vi "Sample Pad Example (LINX).vi"() -> ()   [LabVIEW 2020]
doc: "A simple sample pad, which can trigger up to 16 simultaneous sound effects. Demonstrates the Mixer component, including file loading, playback, and mixer audio monitoring via a music visualizer."
uses:
  Mixer/Channel/Controls/Channel State.ctl
  Mixer/Mixer/Mixer.lvclass/Mixer.ctl
  <vilib>/MakerHub/LINX/Public/Peripherals/Digital/Digital Read N Chans.vi
  e8fa8eb6-c38c-4b8a-b362-922d187964a0.vi
  <vilib>/MakerHub/LINX/Private/Local IO/LinxDigitalRead.vi
  <vilib>/MakerHub/LINX/Public/Utilities/Check Channel.vi
  <vilib>/MakerHub/LINX/Public/Utilities/Open Serial.vi
  <vilib>/MakerHub/LINX/Private/Utilties/Generate Error.vi
  Mixer/Mixer/Polymorphic VIs/Channel Load (Path).vi
  Mixer/Mixer/Mixer.lvclass
  Mixer/Channel/Channel.lvclass
  <vilib>/MakerHub/LINX/LMH-LINX.lvlib
panel:
  in  "Serial Port":refnum<visa-resource-name>="COM3"
  in  "Visualizer":bool
  in  "Sample Path":path
  in  "Stop":bool
  in  "Play 4":bool caption="V"
  in  "Play 3":bool caption="C"
  in  "Play 2":bool caption="X"
  in  "Play 1":bool caption="Z"
  in  "Play 8":bool caption="F"
  in  "Play 7":bool caption="D"
  in  "Play 6":bool caption="S"
  in  "Play 5":bool caption="A"
  in  "Play 12":bool caption="R"
  in  "Play 11":bool caption="E"
  in  "Play 10":bool caption="W"
  in  "Play 9":bool caption="Q"
  in  "Play 16":bool caption="4"
  in  "Play 15":bool caption="3"
  in  "Play 14":bool caption="2"
  in  "Play 13":bool caption="1"
  # "Instructions:\n1. Run the VI.\n2. Select a Sample Path which contains multiple audio files.\n3. Click a button or press the corresponding keyboard key to\n    play the audio sample.\n4. Samples can be played simultaneously, or retriggered by\n    pressing the same button / key in quick succession."
  # "G"
  # "-Audio"
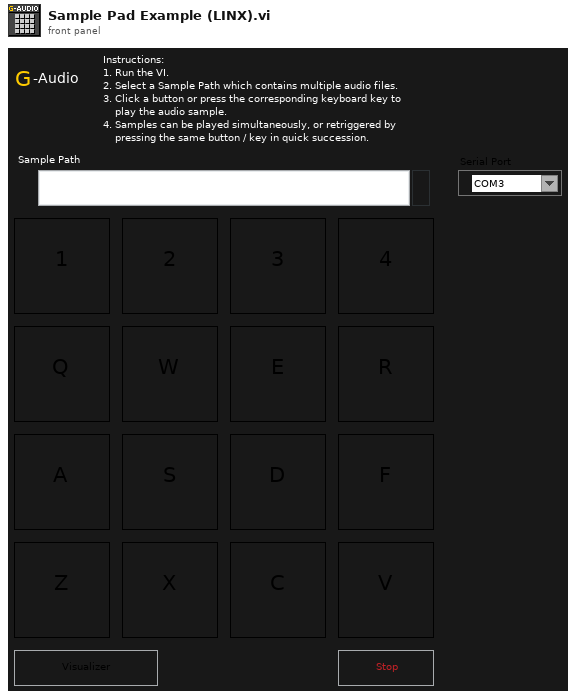
[diagram p1: front panel]
types:
  T1 = typedef "G-Audio.lvlib/Channel.lvclass/Channel State.ctl" = enum16{"Empty", "Error", "Loading", "Loaded", "Stopped", "Paused", "Playing", "Retrigger"}
  T2 = typedef "LMH-LINX.lvlib/LINX Ref.ctl" = cluster{"IO":T3, "Interface":T4, "LINX Device Config":T5}
  T3 = typedef "LMH-LINX.lvlib/Platform.ctl" = enum16{"Remote", "Local"}
  T4 = typedef "LMH-LINX.lvlib/Interface.ctl" = enum16{"Serial", "TCP"}
  T5 = typedef "LMH-LINX.lvlib/Device.lvlib/LINX Device Config.ctl" = cluster{"Interface":T4, "COM Port":refnum<visa-resource-name>, "TCP Configuration":T6, "Device Family":u8, "Device ID":u8, "Device Name":string, "TCP Ref":refnum<k5>, "Channels":T7}
  T6 = typedef "LMH-LINX.lvlib/Device.lvlib/TCP Config.ctl" = cluster{"IP Address":string, "Port":u16}
  T7 = typedef "LMH-LINX.lvlib/Channels.ctl" = cluster{"DI":u8[], "DO":u8[], "AI":u8[], "AO":u8[], "PWM":u8[], "QE":u8[], "UART":u8[], "I2C 2":u8[], "SPI":u8[], "CAN":u8[], "Servo":u8[], "AI Ref (V)":dbl, "AI Resolution (Bits)":u8, "AO Ref (V)":dbl, "AO Resolution (Bits)":u8}
  T8 = enum32{"Invalid", "Standard", "Closed", "Hidden", "Minimized", "Maximized"}
  T9 = typedef "G-Audio.lvlib/Channel.lvclass/Channel Status.ctl" = cluster{"Frame":u64, "State":T1, "Volume":dbl}
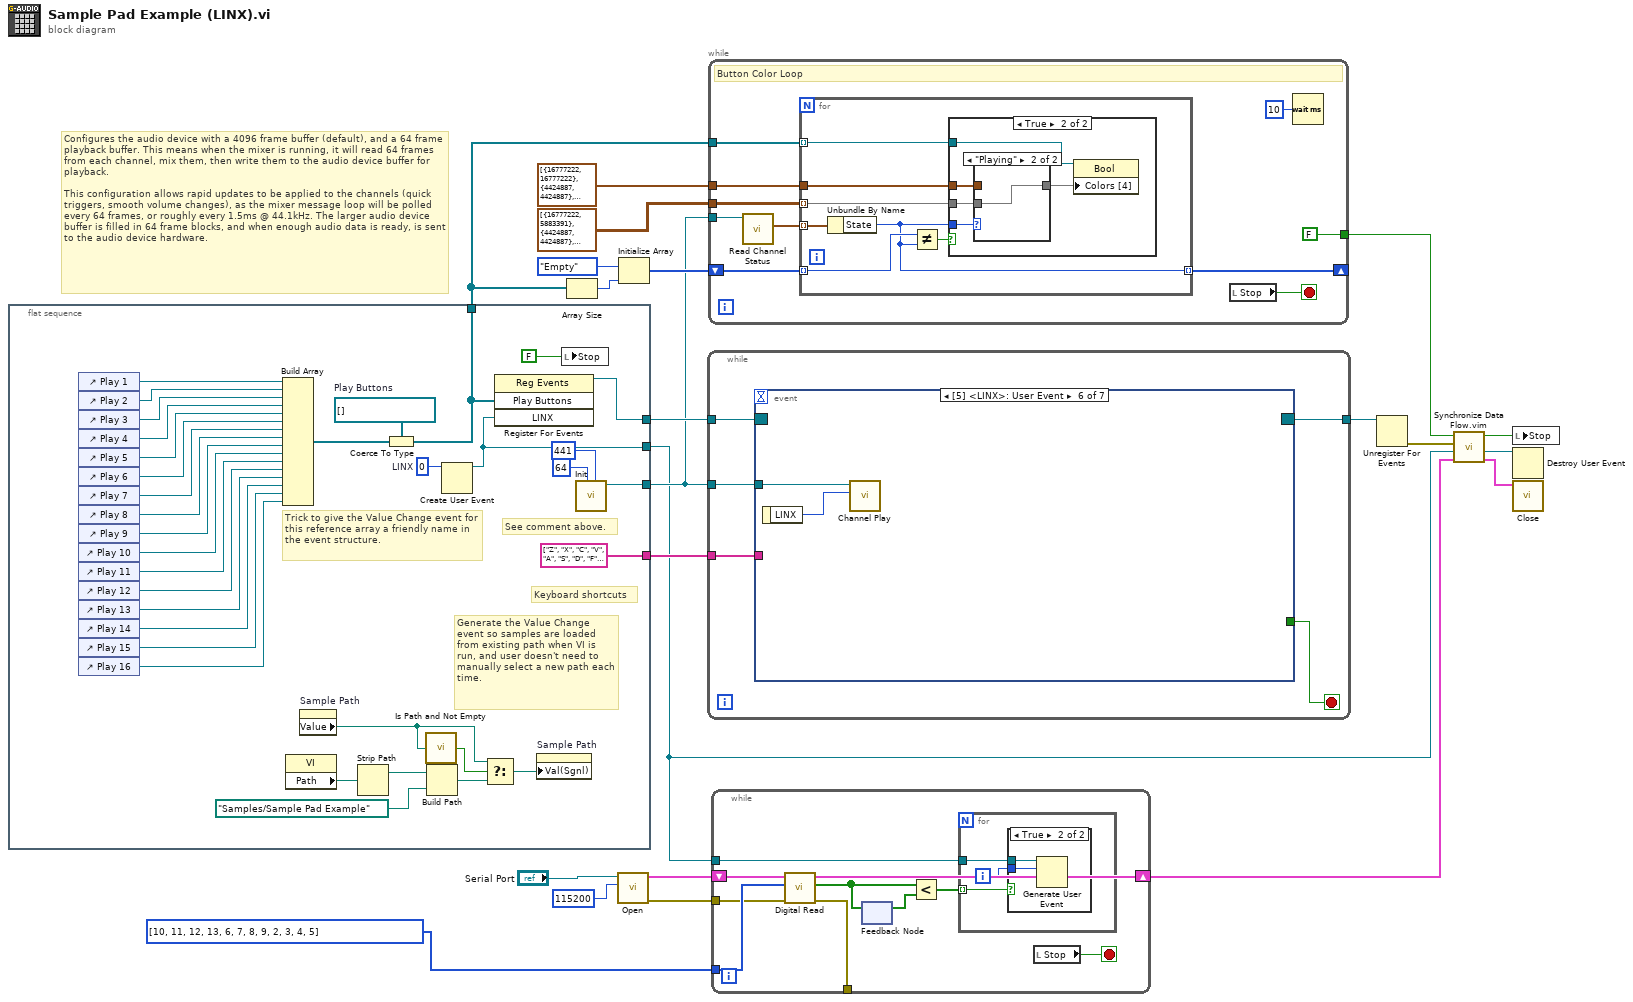
[diagram p0: block diagram]
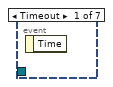
[diagram p5: hidden frame]
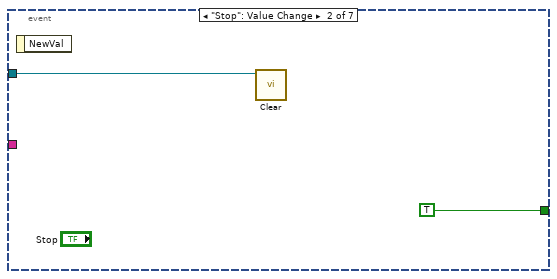
[diagram p6: hidden frame]
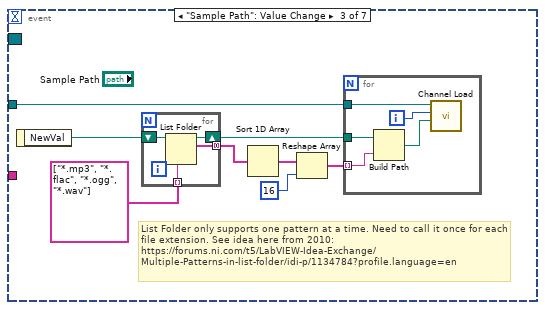
[diagram p7: hidden frame]
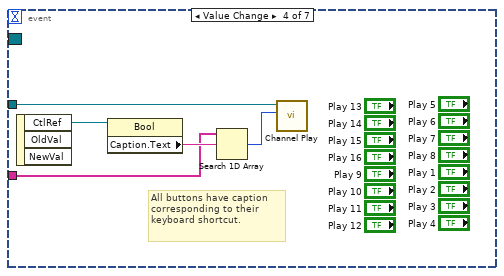
[diagram p8: hidden frame]
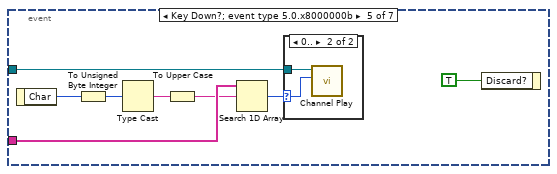
[diagram p9: hidden frame]
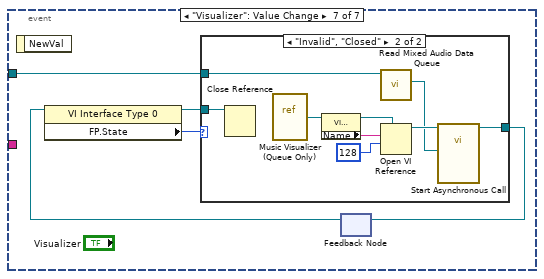
[diagram p11: hidden frame]
diagram:
  # "Configures the audio device with a 4096 frame buffer (default), and a 64 frame playback buffer. This means when the mixer is running, it will read 64 frames from each channel, mix them, then write them to the audio device buffer for playback.\n\nThis configuration allows rapid updates to be applied to the channels (quick triggers, smooth volume changes), as the mixer message loop will be polled every 64 frames, or roughly every 1.5ms @ 44.1kHz. The larger audio device buffer is filled in 64 frame blocks, and when enough audio data is ready, is sent to the audio device hardware."
  n1 = flat-sequence {
    tunnel: [w55] -> w21
    tunnel: [string[] ["Z", "X", "C", "V", "A", "S", "D", "F", "Q", "W", "E", "R", "1", "2", "3", "4"]] -> w20
    tunnel: [w26] -> w11
    tunnel: [w53] -> w14
    tunnel: [w24] -> w4
    frame #0 {
      w25 = 0  # LINX
      w56 = refnum<vi>[] []  # Play Buttons
      # "Trick to give the Value Change event for this reference array a friendly name in the event structure."
      # "See comment above."
      # "Generate the Value Change event so samples are loaded from existing path when VI is run, and user doesn't need to manually select a new path each time."
      # "Keyboard shortcuts"
      n2 = control-ref of="Play 1"() -> (w50:refnum<vi>)
      n3 = control-ref of="Play 2"() -> (w49:refnum<vi>)
      n4 = control-ref of="Play 3"() -> (w48:refnum<vi>)
      n5 = control-ref of="Play 4"() -> (w47:refnum<vi>)
      n6 = control-ref of="Play 5"() -> (w46:refnum<vi>)
      n7 = control-ref of="Play 6"() -> (w45:refnum<vi>)
      n8 = control-ref of="Play 7"() -> (w44:refnum<vi>)
      n9 = control-ref of="Play 8"() -> (w43:refnum<vi>)
      n10 = control-ref of="Play 9"() -> (w42:refnum<vi>)
      n11 = control-ref of="Play 10"() -> (w41:refnum<vi>)
      n12 = control-ref of="Play 11"() -> (w40:refnum<vi>)
      n13 = control-ref of="Play 12"() -> (w39:refnum<vi>)
      n14 = control-ref of="Play 13"() -> (w38:refnum<vi>)
      n15 = control-ref of="Play 14"() -> (w37:refnum<vi>)
      n16 = control-ref of="Play 15"() -> (w36:refnum<vi>)
      n17 = control-ref of="Play 16"() -> (w35:refnum<vi>)
      n18 = Build Array(w50, w49, w48, w47, w46, w45, w44, w43, w42, w41, w40, w39, w38, w37, w36, w35) -> (w51:refnum<vi>[])
      n19 = property class="VI"() -> ("Path"=w32:path)  [unwired: 2 in, 2 out]
      n20 = property on="Sample Path" class="Path"() -> ("Value"=w28:path)  [unwired: 2 in, 2 out]
      n21 = Strip Path(path=w32) -> (stripped path=w31:path)  [unwired: 1 out]
      n22 = Coerce To Type(0:w51, 1:w56) -> (2:w26:refnum<vi>[])
      n23 = call <vilib>:"Is Path and Not Empty.vi"("path"=w28) -> ("Is Path and Not Empty?"=w34:bool)  [unwired: 4 in]
      n24 = Build Path(base path=w31, name or relative path=path "Samples/Sample Pad Example") -> (appended path=w29:path)
      n25 = Create User Event(user event datatype=w25) -> (user event=w24:refnum<user-event>)  [unwired: 1 in, 1 out]
      n26 = Select(t=w28, s=w34, f=w29) -> (s? t:f=w33:path)
      n27 = register-events(w26, w24) -> (reference out=w55:refnum<event-registration>)  [unwired: 2 in, 1 out]
      n28 = property on="Sample Path" class="Path"("Val(Sgnl)"=w33) -> ()  [unwired: 2 in, 2 out]
      n29 = local write "Stop"(FALSE ("Stop")) -> ()
      n30 = call "Init.vi"("Buffer Size (4096)"=441, "Playback Size (4096)"=64) -> ("Mixer out"=w53:refnum<class "Mixer.lvclass">)  [unwired: 8 in, 1 out]
    }
  }
  n31 = Array Size(array=w11) -> (size(s)=w12:i32)
  n32 = call-poly <vilib>:"Open.vi"("Baud Rate Override"=u32 115200, "Serial Port"="Serial Port") -> ("Error Out"=w2:errorcluster, "LINX Resource"=w10:T2)  [unwired: 7 in, 1 out]
  n33 = Initialize Array(Channel_State."Empty" ("State"), w12) -> (w22:T1[])
  n34 = while {
    tunnel: w21 -> [w61]
    tunnel: w14 -> [w60]
    tunnel: w20 -> [w59]
    tunnel: [w57] -> w19
    stop <- w58 stop-if-true
    n35 = event shown="[5] <LINX>: User Event" {
      selector: w61 -> [_ _ _ _ _ _ _]
      dyn-events: [_ _ _ _ _ _ _] -> w57
      timeout: _ -> [_ _ _ _ _ _ _]
      tunnel: w60 -> [_ w63 w69 w84 w93 w97 w101]
      tunnel: w59 -> [_ _ _ w82 w91 _ _]
      tunnel: [_ TRUE _ _ _ _ _] -> w58
      event Timeout {
        n36 = event-data() -> ()  [unwired: 1 in, 1 out]
      }
      event "Stop": Value Change {
        n37 = event-data() -> ()  [unwired: 1 in, 1 out]
        n38 = call "Clear.vi"("Mixer in"=w63) -> ()  [unwired: 10 in, 1 out]
      }
      event "Sample Path": Value Change {
        # "List Folder only supports one pattern at a time. Need to call it once for each file extension. See idea here from 2010:\nhttps://forums.ni.com/t5/LabVIEW-Idea-Exchange/Multiple-Patterns-in-list-folder/idi-p/1134784?profile.language=en"
        n39 = event-data() -> ("NewVal"=w64:path)  [unwired: 1 in]
        n40 = for {
          shift-right: [w75] -> w70
          shift-left: w64 -> [w74]
          tunnel: string[] ["*.mp3", "*.flac", "*.ogg", "*.wav"] -> [w73] mode=indexing
          tunnel: [w72] -> w66 mode=concatenating
          n41 = List Folder(path=w74, pattern=w73) -> (path out=w75:path, filenames=w72:string[])  [unwired: 2 in, 2 out]
        }
        n42 = Sort 1D Array(array=w66) -> (sorted array=w65:string[])
        n43 = Reshape Array(w65, 16 ("dimension size")) -> (w71:string[])
        n44 = for {
          tunnel: w71 -> [w80] mode=indexing
          tunnel: w70 -> [w79]
          tunnel: w69 -> [w78]
          i -> [w77]
          n45 = Build Path(base path=w79, name or relative path=w80) -> (appended path=w76:path)
          n46 = call-poly "Channel Load.vi"("Path"=w76, "Channel Index"=w77, "Mixer in"=w78) -> ()  [unwired: 7 in, 2 out]
        }
      }
      event Value Change {
        # "All buttons have caption corresponding to their keyboard shortcut."
        n47 = event-data() -> ("CtlRef"=w85:refnum<vi>)  [unwired: 1 in, 2 out]
        n48 = property class="Bool"(reference=w85) -> ("Caption.Text"=w83:string)  [unwired: 1 in, 2 out]
        n49 = Search 1D Array(1D array=w82, element=w83) -> (index of element=w81:i32)  [unwired: 1 in]
        n50 = call "Channel Play.vi"("Channel Index"=w81, "Mixer in"=w84) -> ()  [unwired: 8 in, 2 out]
      }
      event Key Down?; event type 5.0.x8000000b {
        n51 = event-data() -> ("Char"=w92:i16)  [unwired: 1 in]
        n52 = To Unsigned Byte Integer(number=w92) -> (unsigned 8bit integer=w88:u8)
        n53 = Type Cast(x=w88) -> (*(type *) &x=w86:string)  [unwired: 1 in]
        n54 = To Upper Case(1:w86) -> (0:w89:string)
        n55 = Search 1D Array(1D array=w91, element=w89) -> (index of element=w87:i32)  [unwired: 1 in]
        n56 = case shown="0.." w87 {
          selector: w87 -> [_ w94]
          tunnel: w93 -> [_ w95]
          frame Default {
          }
          frame 0.. {
            n57 = call "Channel Play.vi"("Channel Index"=w94, "Mixer in"=w95) -> ()  [unwired: 8 in, 2 out]
          }
        }
        n58 = event-data("Discard?"=TRUE) -> ()  [unwired: 1 in, 1 out]
      }
      event User Event {
        n59 = event-data() -> ("LINX"=w96:i32)  [unwired: 1 in]
        n60 = call "Channel Play.vi"("Channel Index"=w96, "Mixer in"=w97) -> ()  [unwired: 8 in, 2 out]
      }
      event "Visualizer": Value Change {
        n61 = event-data() -> ()  [unwired: 1 in, 1 out]
        n62 = feedback #1() -> (w98:refnum<vi>)  [unwired: 1 in]
        n63 = property class="VI Interface Type 0"(reference=w98) -> (reference out=w100:refnum<vi>, "FP.State"=w99:T8)  [unwired: 1 in, 1 out]
        n64 = case shown="\"Invalid\", \"Closed\"" w99 {
          tunnel: [w103 w107] -> w102
          tunnel: w101 -> [_ w106]
          tunnel: w100 -> [w103 w104]
          frame Default {
          }
          frame "Invalid", "Closed" {
            n65 = Close Reference(reference=w104) -> ()  [unwired: 1 in, 1 out]
            n66 = vi-ref "Music Visualizer (Queue Only).vi"() -> (w112:refnum<vi>)
            n67 = property class="VI (strict)"(reference=w112) -> (reference out=w110:refnum<vi>, "Name"=w111:string)  [unwired: 1 in, 1 out]
            n68 = call "Read Mixed Audio Data Queue.vi"("Mixer in"=w106) -> ("Mixed Audio Data"=w105:refnum<queue>)  [unwired: 8 in, 2 out]
            n69 = Open VI Reference(type specifier VI Refnum (for type only)=w110, vi path=w111, options=128) -> (vi reference=w108:refnum<vi>)  [unwired: 3 in, 1 out]
            n70 = call-by-ref "Start Asynchronous Call"(reference=w108, "Mixed Audio Data"=w105) -> (reference out=w107:refnum<vi>)  [unwired: 12 in, 1 out]
          }
        }
        n71 = feedback-in #1(w102) -> ()
      }
    }
  }
  n72 = while {
    tunnel: w14 -> [w122]
    tunnel: w11 -> [w120]
    tunnel: cluster{u32, u32}[] [{16777222, 16777222}, {4424887, 4424887}, {4424887, 4424887}, {4424887, 4424887}] ("Colors [4]") -> [w119]
    tunnel: cluster{"Color Box":u32, "Color Box":u32}[][] [[{"Color Box"=16777222, "Color Box"=5883391}, {"Color Box"=4424887, "Color Box"=4424887}, {"Color Box"=4424887, "Color Box"=4424887}, {"Color Box"=4424887, "Color Box"=4424887}], [{"Color Box"=16777222, "Color Box"=5883391}, {"Color Box"=4424887, "Color Box"=4424887}, {"Color Box"=4424887, "Color Box"=4424887}, {"Color Box"=4424887, "Color Box"=4424887}], [{"Color Box"=16777222, "Color Box"=5883391}, {"Color Box"=4424887, "Color Box"=4424887}, {"Color Box"=4424887, "Color Box"=4424887}, {"Color Box"=4424887, "Color Box"=4424887}], [{"Color Box"=16777222, "Color Box"=5883391}, {"Color Box"=4424887, "Color Box"=4424887}, {"Color Box"=4424887, "Color Box"=4424887}, {"Color Box"=4424887, "Color Box"=4424887}], [{"Color Box"=16777222, "Color Box"=6618880}, {"Color Box"=4424887, "Color Box"=4424887}, {"Color Box"=4424887, "Color Box"=4424887}, {"Color Box"=4424887, "Color Box"=4424887}], [{"Color Box"=16777222, "Color Box"=6618880}, {"Color Box"=4424887, "Color Box"=4424887}, {"Color Box"=4424887, "Color Box"=4424887}, {"Color Box"=4424887, "Color Box"=4424887}], [{"Color Box"=16777222, "Color Box"=6618880}, {"Color Box"=4424887, "Color Box"=4424887}, {"Color Box"=4424887, "Color Box"=4424887}, {"Color Box"=4424887, "Color Box"=4424887}], [{"Color Box"=16777222, "Color Box"=6618880}, {"Color Box"=4424887, "Color Box"=4424887}, {"Color Box"=4424887, "Color Box"=4424887}, {"Color Box"=4424887, "Color Box"=4424887}], [{"Color Box"=16777222, "Color Box"=16746514}, {"Color Box"=4424887, "Color Box"=4424887}, {"Color Box"=4424887, "Color Box"=4424887}, {"Color Box"=4424887, "Color Box"=4424887}], [{"Color Box"=16777222, "Color Box"=16746514}, {"Color Box"=4424887, "Color Box"=4424887}, {"Color Box"=4424887, "Color Box"=4424887}, {"Color Box"=4424887, "Color Box"=4424887}], [{"Color Box"=16777222, "Color Box"=16746514}, {"Color Box"=4424887, "Color Box"=4424887}, {"Color Box"=4424887, "Color Box"=4424887}, {"Color Box"=4424887, "Color Box"=4424887}], [{"Color Box"=16777222, "Color Box"=16746514}, {"Color Box"=4424887, "Color Box"=4424887}, {"Color Box"=4424887, "Color Box"=4424887}, {"Color Box"=4424887, "Color Box"=4424887}], [{"Color Box"=16777222, "Color Box"=16711680}, {"Color Box"=4424887, "Color Box"=4424887}, {"Color Box"=4424887, "Color Box"=4424887}, {"Color Box"=4424887, "Color Box"=4424887}], [{"Color Box"=16777222, "Color Box"=16711680}, {"Color Box"=4424887, "Color Box"=4424887}, {"Color Box"=4424887, "Color Box"=4424887}, {"Color Box"=4424887, "Color Box"=4424887}], [{"Color Box"=16777222, "Color Box"=16711680}, {"Color Box"=4424887, "Color Box"=4424887}, {"Color Box"=4424887, "Color Box"=4424887}, {"Color Box"=4424887, "Color Box"=4424887}], [{"Color Box"=16777222, "Color Box"=16711680}, {"Color Box"=4424887, "Color Box"=4424887}, {"Color Box"=4424887, "Color Box"=4424887}, {"Color Box"=4424887, "Color Box"=4424887}]] ("appended array") -> [w118]
    tunnel: [FALSE ("Stop")] -> w16
    shift-right: [w114] -> _
    shift-left: w22 -> [w113]
    stop <- w116 stop-if-true
    # "Button Color Loop"
    n73 = call "Read Channel Status.vi"("Mixer in"=w122) -> ("Channel Status"=w121:T9[])  [unwired: 8 in, 2 out]
    n74 = for {
      tunnel: w121 -> [w129] mode=indexing
      tunnel: w120 -> [w128] mode=indexing
      tunnel: w119 -> [w127]
      tunnel: w118 -> [w126] mode=indexing
      tunnel: [w123] -> w114 mode=indexing
      tunnel: w113 -> [w125] mode=indexing
      n75 = Unbundle By Name(w129) -> ("State"=w123:T1)
      n76 = Not Equal?(x=w125, y=w123) -> (x != y?=w124:bool)
      n77 = case shown="True" w124 {
        tunnel: w128 -> [_ w134]
        tunnel: w127 -> [_ w133]
        tunnel: w126 -> [_ w131]
        tunnel: w123 -> [_ w130]
        frame False {
        }
        frame True {
          n78 = case shown="\"Playing\"" w130 {
            tunnel: w133 -> [w135 _]
            tunnel: [w135 w136] -> w132
            tunnel: w131 -> [_ w136]
            frame Default {
            }
            frame "Playing" {
            }
          }
          n79 = property class="Bool"(reference=w134, "Colors [4]"=w132) -> ()  [unwired: 1 in, 2 out]
        }
      }
    }
    n80 = local read "Stop"() -> (w116:bool)
    n81 = Wait (ms)(milliseconds to wait=u32 10) -> ()  [unwired: 1 out]
  }
  n82 = while {
    tunnel: u8[] [10, 11, 12, 13, 6, 7, 8, 9, 2, 3, 4, 5] -> [w145]
    tunnel: w4 -> [w141]
    shift-right: [w140] -> w6
    shift-left: w10 -> [w146]
    tunnel: w2 -> [w138]
    tunnel: [w137] -> _
    stop <- w139 stop-if-true
    n83 = call-poly <vilib>:"Digital Read.vi"("Error In"=w138, "DI Channels"=w145, "LINX Resource"=w146) -> ("Error Out"=w137:errorcluster, "Values"=w144:bool[], "LINX Resource"=w140:T2)  [unwired: 6 in]
    n84 = feedback-in #2(w144) -> ()
    n85 = feedback #2() -> (w143:bool[])  [unwired: 1 in]
    n86 = Less?(x=w144, y=w143) -> (x < y?=w142:bool[])
    n87 = for {
      tunnel: w142 -> [w148] mode=indexing
      tunnel: w141 -> [w149]
      i -> [w147]
      n88 = case shown="True" w148 {
        tunnel: w149 -> [_ w151]
        tunnel: w147 -> [_ w150]
        frame False {
        }
        frame True {
          n89 = Generate User Event(user event=w151, event data cluster=w150) -> ()  [unwired: 2 in, 2 out]
        }
      }
    }
    n90 = local read "Stop"() -> (w139:bool)
  }
  n91 = Unregister For Events(event registration refnum=w19) -> (error out=w7:errorcluster)  [unwired: 1 in]
  n92 = call "Synchronize Data Flow.vim"("input 4"=w6, "input 3"=w4, "input 2"=w7, "input 1"=w16) -> ("output 4"=w5:T2, "output 3"=w3:refnum<user-event>, "output 1"=w17:bool)  [unwired: 1 out]
  n93 = local write "Stop"(w17) -> ()
  n94 = Destroy User Event(user event=w3) -> ()  [unwired: 1 in, 1 out]
  n95 = call <vilib>:"Close.vi"("LINX Resource"=w5) -> ()  [unwired: 10 in, 1 out]
